vi "RT_velocity_plus.vi"() -> ()   [LabVIEW 2014]
uses:
  <vilib>/FPGAPlugInAG/cRIO-9068/niLvFpga_Open_cRIO-9068.vi
  <vilib>/rvi/interface/common/dynamic/niFpgaDynamicAddResources.vi
  <vilib>/Utility/error.llb/Error Cluster From Error Code.vi
  <vilib>/rvi/errors/niLvFpgaAdjustHostInterfaceError.vi
  <vilib>/FPGAPlugInAG/Dynamic/niLvFpga_Close_Dynamic.vi
  <vilib>/rvi/interface/nirviOpenFPGA/nirviOpenFPGA.xnode
  FPGA Bitfiles/Motortest_FPGATarget_test6auto_Jx62XASY7Q8.lvbitx
  <vilib>/rvi/interface/nirviReadWriteControl/nirviReadWriteControl.xnode
  <vilib>/rvi/interface/nirviCloseFPGA/nirviCloseFPGA.xnode
  NiFpgaLv.dll
  <vilib>/rvi/interface/Simulation/niFpgaSimulationCallBeginRW.vi
panel:
  out "Velocity":cluster{i32[], sgl[]}(graph)
  in  "Desired Velocity [Round/s]":dbl
  out "Position":cluster{i32[], sgl[]}(graph)
  out "Position[Round]":sgl
  out "Angular Velocity vs. Duty Cycle":cluster{dbl[], sgl[]}(graph)
  in  "Drive Direction":enum8{"Clockwise", "Counterclockwise"}(ring)=enum."Counterclockwise"
  in  "Velocity Interval (uSec)":u32=500000
  in  "stop":bool
  out "Velocity[RPS]":sgl
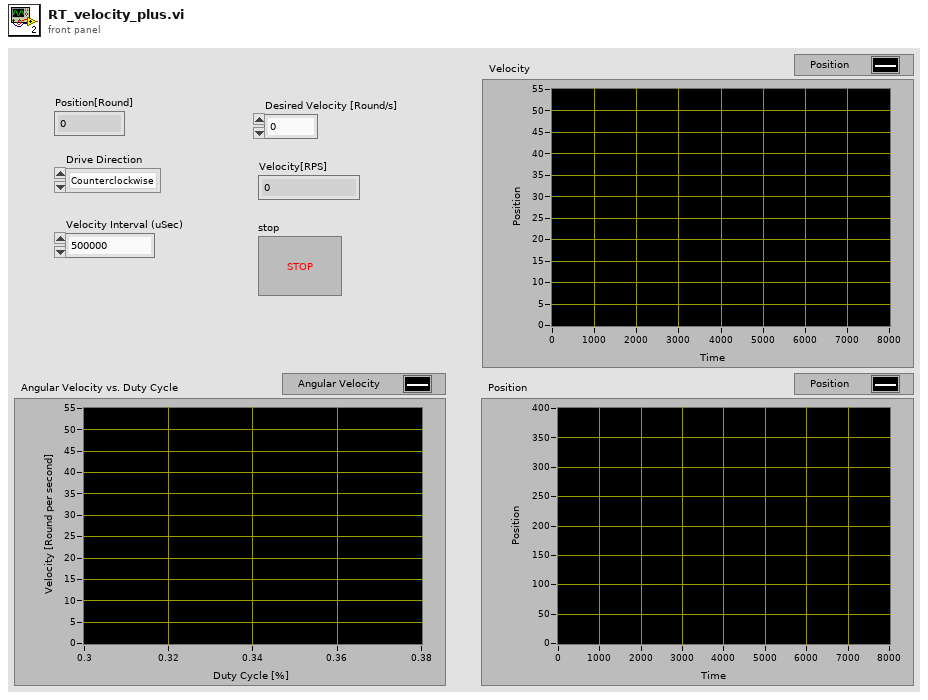
[diagram p1: front panel]
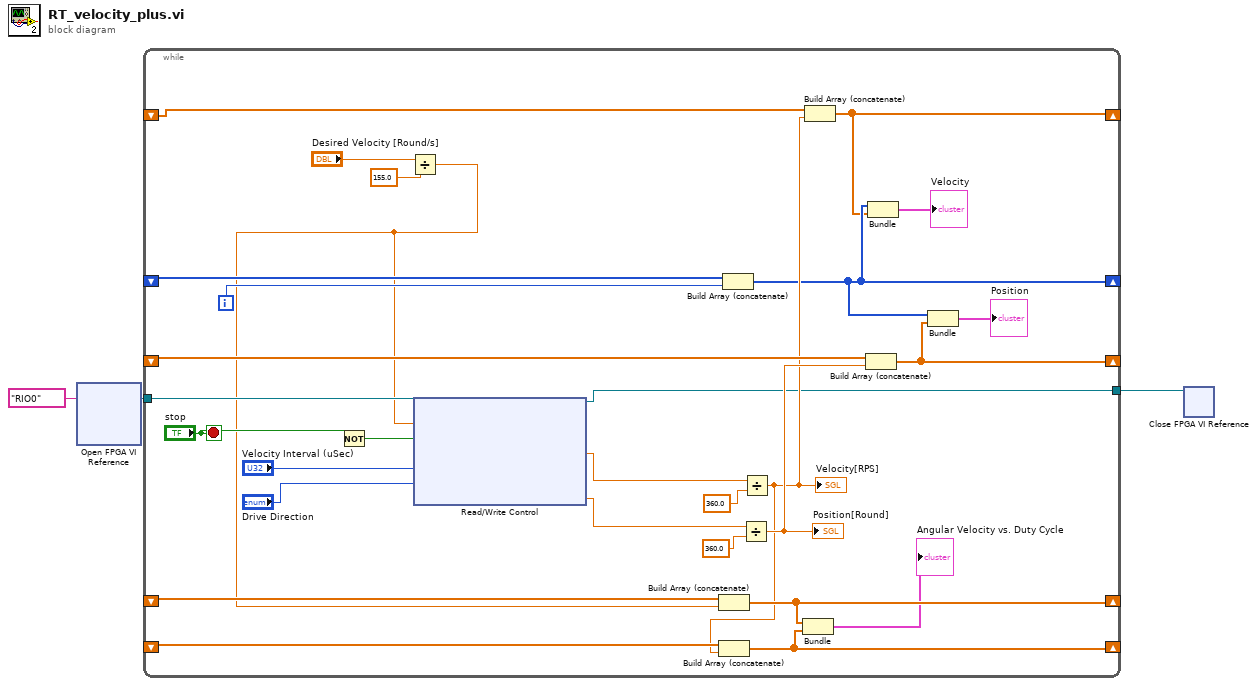
[diagram p0: block diagram]
diagram:
  n1 = xnode "Open FPGA VI Reference"("resource name"=tag "RIO0") -> ("FPGA VI Reference Out"=w2:refnum<k20>)  [unwired: 1 in, 1 out]
  n2 = while {
    tunnel: w2 -> [w11]
    shift-right: [w31] -> _
    shift-left: _ -> [w20]
    shift-right: [w25] -> _
    shift-left: _ -> [w21]
    shift-right: [w13] -> _
    shift-left: _ -> [w26]
    shift-right: [w23] -> _
    shift-left: _ -> [w24]
    shift-right: [w12] -> _
    shift-left: _ -> [w16]
    tunnel: [w5] -> w1
    i -> [w27]
    stop <- "stop" stop-if-true
    n3 = Not(x="stop") -> (.not. x?=w10:bool)
    n4 = Divide(x="Desired Velocity [Round/s]", y=155.0) -> (x/y=w4:dbl)
    n5 = xnode "Read/Write Control"("FPGA VI Reference In"=w11, "duty cycle (periods)"=w4, "Mod1/Motor"=w10, "Velocity Interval (uSec)"="Velocity Interval (uSec)", "Mod1/Drive Direction"="Drive Direction") -> ("FPGA VI Reference Out"=w5:refnum<k20>, "Velocity (Degrees/Second)"=w7:sgl, "Position (Degrees)"=w6:sgl)  [unwired: 1 in, 1 out]
    n6 = Build Array (concatenate)(w20, w4) -> (w31:dbl[])
    n7 = Build Array (concatenate)(w26, w27) -> (w13:i32[])
    n8 = Divide(x=w6, y=sgl 360.0) -> (x/y=w19:sgl)
    "Position[Round]" <- w19
    n9 = Divide(x=w7, y=sgl 360.0) -> (x/y=w15:sgl)
    "Velocity[RPS]" <- w15
    n10 = Build Array (concatenate)(w21, w15) -> (w25:sgl[])
    n11 = Bundle(w31, w25) -> (→"Angular Velocity vs. Duty Cycle":cluster{dbl[], sgl[]})  [unwired: 1 in]
    n12 = Build Array (concatenate)(w16, w15) -> (w12:sgl[])
    n13 = Build Array (concatenate)(w24, w19) -> (w23:sgl[])
    n14 = Bundle(w13, w12) -> (→"Velocity":cluster{i32[], sgl[]})  [unwired: 1 in]
    n15 = Bundle(w13, w23) -> (→"Position":cluster{i32[], sgl[]})  [unwired: 1 in]
  }
  n16 = xnode "Close FPGA VI Reference"("FPGA VI Reference In"=w1) -> ()  [unwired: 1 in, 1 out]
